vi "New TCP Socket Server.vi"(6 "log service":refnum<data-value>, 7 "max connections (-1:unlimited)":i32=-1, 8 "error in (no error)":errorcluster, 9 "Connection Handler":refnum<class "Connection Handler.lvclass">, 10 "port":u16, 11 "servvice name":string) -> (0 "error out":errorcluster, 3 "TCP Server":refnum<data-value>)   [LabVIEW 2019, in "TCP Socket Server.lvclass"]
uses:
  TCP Socket Server.lvclass
  Connection Handler/Connection Handler.lvclass
  TCP Socket Server.lvclass/TCP Socket Server.ctl
  a0a41830-1a45-43cf-bd2a-015309dc2ff0.vi
  Enumerating Connection Hanlder/Enumerating Connection Handler.lvclass
  C:/Users/Nicholas Folse/Documents/workspace/github-tauterra.llc/ANODE/ANODE/Socket API/Connection Handler/Connection Handler.lvclass
  subVIs/tcp_server_monitor.vi
  Utility API/Log Service/Log Service.lvclass
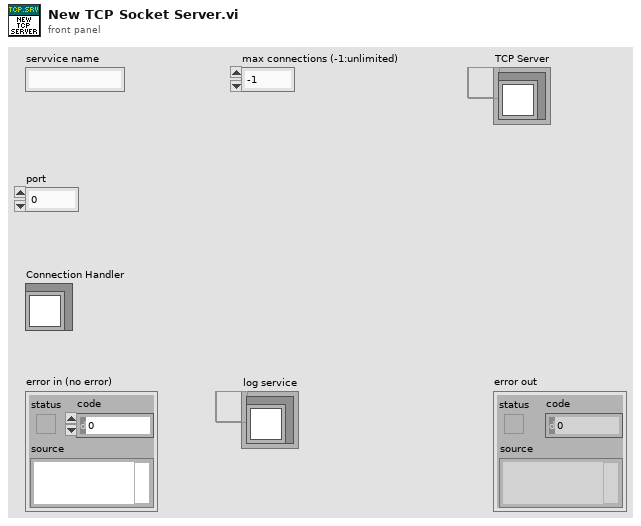
[diagram p1: front panel]
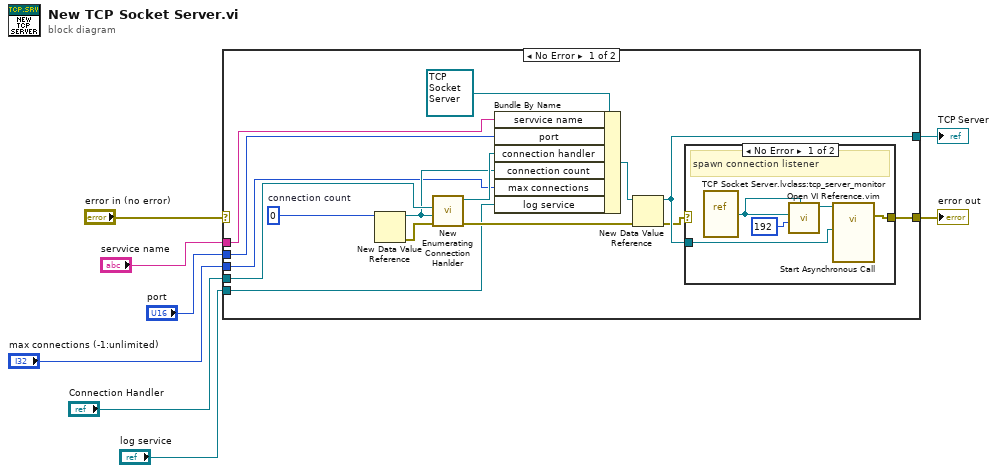
[diagram p0: block diagram]
diagram:
  n1 = case shown="No Error" "error in (no error)" {
    selector: "error in (no error)" -> [_ w30]
    tunnel: "Connection Handler" -> [w16 _]
    tunnel: "servvice name" -> [w22 _]
    tunnel: "port" -> [w21 _]
    tunnel: [w19 _] -> w4
    tunnel: [w17 w30] -> w3
    tunnel: "max connections (-1:unlimited)" -> [w10 _]
    tunnel: "log service" -> [w9 _]
    frame No Error {
      w14 = 0  # connection count
      n2 = New Data Value Reference(data value=w14) -> (data value reference=w13:refnum<data-value>, error out=w12:errorcluster)  [unwired: 1 in]
      n3 = call "New Enumerating Connection Hanlder.vi"("error in (no error)"=w12, "connection count"=w13, "Connection Handler"=w16) -> ("error out"=w11:errorcluster, "Enumerating Connection Handler out"=w15:refnum<class "Enumerating Connection Handler.lvclass">)  [unwired: 7 in]
      n4 = Bundle By Name(cluster=refnum<class "TCP Socket Server.lvclass"> refnum ("TCP Socket Server in"), "servvice name"=w22, "port"=w21, "connection handler"=w15, "connection count"=w13, "max connections"=w10, "log service"=w9) -> (w20:refnum<class "TCP Socket Server.lvclass">)
      n5 = New Data Value Reference(data value=w20, error in=w11) -> (data value reference=w19:refnum<data-value>, error out=w18:errorcluster)
      n6 = case shown="No Error" w18 {
        selector: w18 -> [_ w29]
        tunnel: w19 -> [w25 _]
        tunnel: [w24 w29] -> w17
        frame No Error {
          # "spawn connection listener"
          n7 = vi-ref "TCP Socket Server.lvclass:tcp_server_monitor.vi"() -> (w27:refnum<vi>)
          n8 = call "Open VI Reference.vim"("type specifier VI Refnum (for type only)"=w27, "options"=192, "vi reference"=w27) -> ("vi reference out"=w26:refnum<vi>)  [unwired: 7 in, 1 out]
          n9 = call-by-ref "Start Asynchronous Call"(reference=w26, "TCP Socket Server in"=w25) -> (error out=w24:errorcluster)  [unwired: 12 in, 1 out]
        }
        frame Error {
        }
      }
    }
    frame Error {
    }
  }
  "error out" <- w3
  "TCP Server" <- w4
